vi "Datasheet Create Table Row.vi"(8 "error in (no error)":errorcluster, 9 "TDM Data":T2[](array[typedef]), 10 "Columns":T1[](array[typedef])) -> (0 "error out":errorcluster, 2 "Comma row":string, 3 "HTM Row":string)   [LabVIEW 2011]
uses:
  TDMS/TDMS File.ctl
  TDMS/TDMS Run.ctl
  TDMS/TDMS Channel (Sxx).ctl
  database/Fields/Field Record.ctl
  database/Fields/Field DataTypes.ctl
  database/Fields/Field NextItem.ctl
  Column Data.ctl
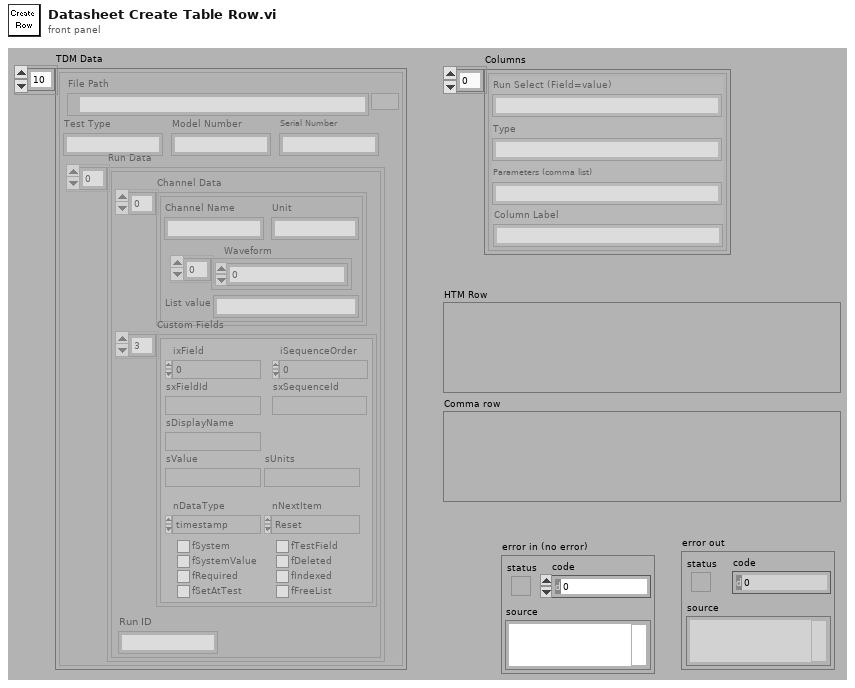
[diagram p1: front panel]
types:
  T1 = typedef "Column Data.ctl" = cluster{"Run Select (Field=value)":string, "Type":string, "Parameters (comma list)":string, "Column Label":string}
  T2 = typedef "TDMS File.ctl" = cluster{"File Path":path, "Run Data":T3[], "Serial Number":string, "Model Number":string, "Test Type":string}
  T3 = typedef "TDMS Run.ctl" = cluster{"Channel Data":T4[], "Custom Fields":T5[], "Run ID":string}
  T4 = typedef "TDMS Channel (Sxx).ctl" = cluster{"Channel Name":string, "Waveform":dbl[], "Unit":string, "List value":string}
  T5 = typedef "Field Record.ctl" = cluster{"ixField":i32, "iSequenceOrder":i32, "sxFieldId":string, "sxSequenceId":string, "sDisplayName":string, "sValue":string, "sUnits":string, "nDataType":T6, "nNextItem":T7, "fSystem":bool, "fSystemValue":bool, "fRequired":bool, "fSetAtTest":bool, "fTestField":bool, "fDeleted":bool, "fIndexed":bool, "fFreeList":bool}
  T6 = typedef "Field DataTypes.ctl" = enum32{"text", "numeric", "list", "timestamp", "boolean"}
  T7 = typedef "Field NextItem.ctl" = enum32{"Reset", "Retain", "Auto-Increment"}
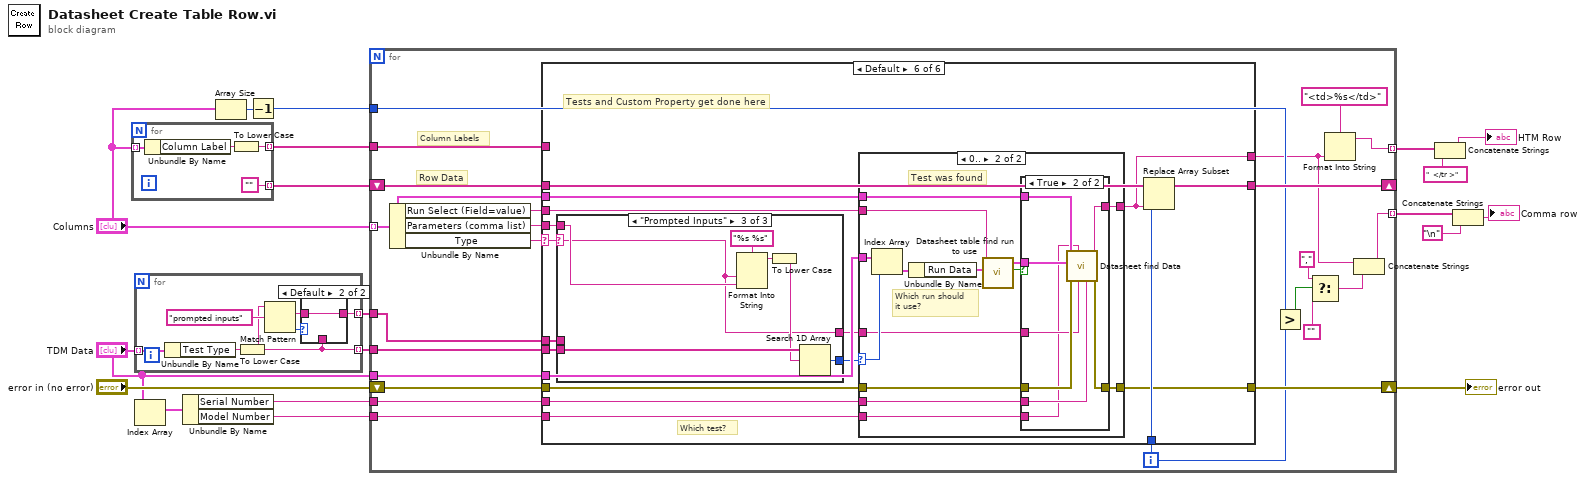
[diagram p0: block diagram]
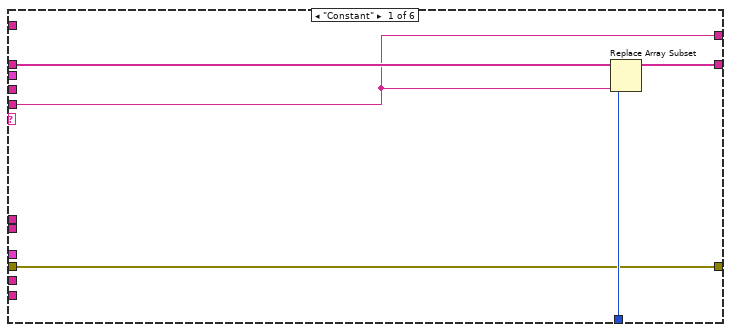
[diagram p3: hidden frame]
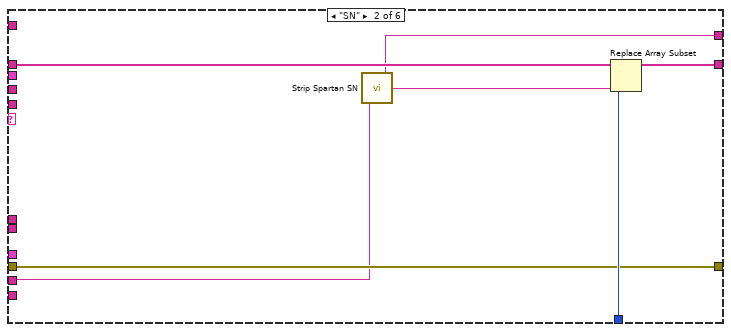
[diagram p4: hidden frame]
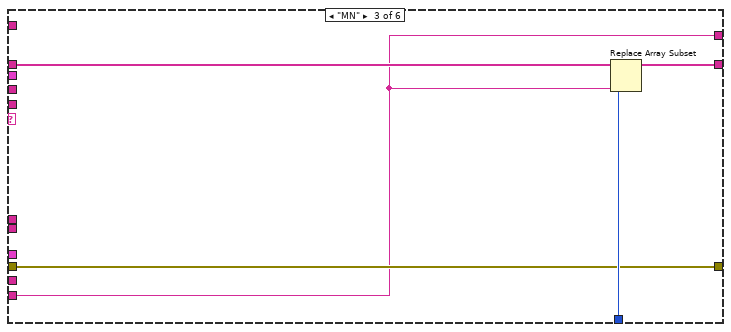
[diagram p5: hidden frame]
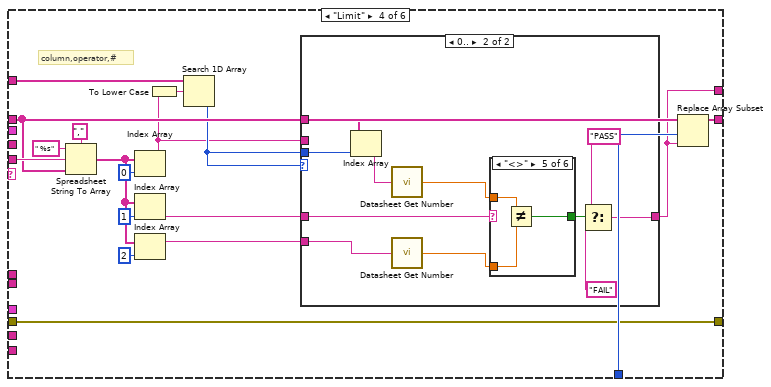
[diagram p6: hidden frame]
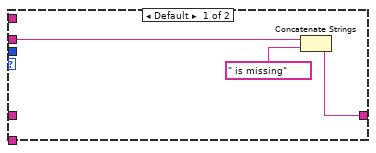
[diagram p7: hidden frame]
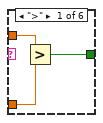
[diagram p8: hidden frame]
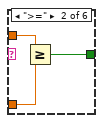
[diagram p9: hidden frame]
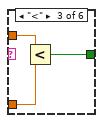
[diagram p10: hidden frame]
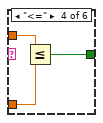
[diagram p11: hidden frame]
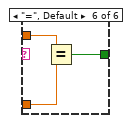
[diagram p12: hidden frame]
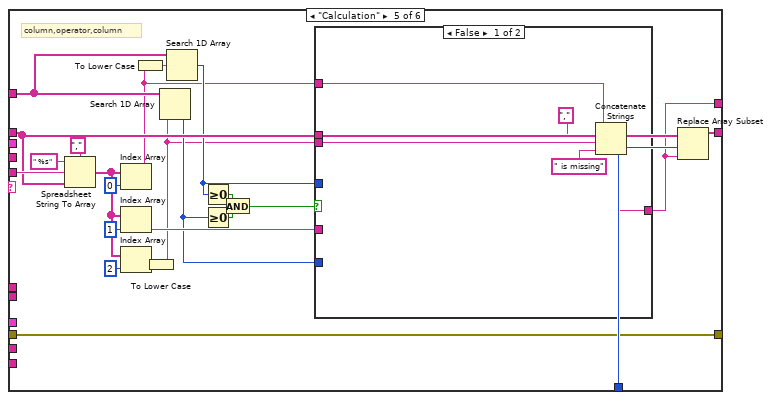
[diagram p13: hidden frame]
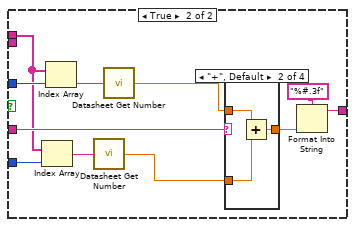
[diagram p14: hidden frame]
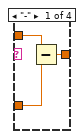
[diagram p15: hidden frame]
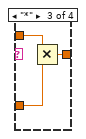
[diagram p16: hidden frame]
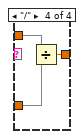
[diagram p17: hidden frame]
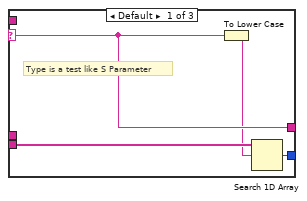
[diagram p18: hidden frame]
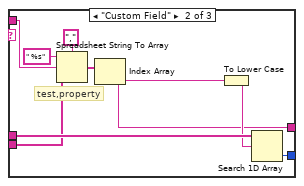
[diagram p19: hidden frame]
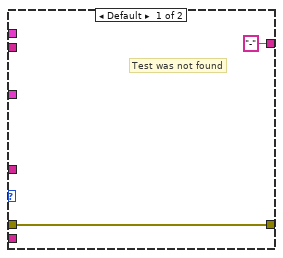
[diagram p20: hidden frame]
diagram:
  n1 = for {
    tunnel: "Columns" -> [w23] mode=indexing
    tunnel: [""] -> w16 mode=indexing
    tunnel: [w20] -> w3 mode=indexing
    n2 = Unbundle By Name(w23) -> ("Column Label"=w21:string)
    n3 = To Lower Case(string=w21) -> (all lower case string=w20:string)
  }
  n4 = for {
    tunnel: "TDM Data" -> [w30] mode=indexing
    tunnel: [w25] -> w17 mode=indexing
    tunnel: [w26] -> w1 mode=indexing
    n5 = Unbundle By Name(w30) -> ("Test Type"=w29:string)
    n6 = To Lower Case(string=w29) -> (all lower case string=w25:string)
    n7 = Match Pattern(string=w25, regular expression="prompted inputs") -> (match substring=w24:string, offset past match=w27:i32)  [unwired: 1 in, 2 out]
    n8 = case shown="Default" w27 {
      tunnel: [w31 w32] -> w26
      tunnel: w25 -> [w31 _]
      tunnel: w24 -> [_ w32]
      frame -1 {
      }
      frame Default {
      }
    }
  }
  n9 = Index Array(array="TDM Data") -> (element=w9:T2)  [unwired: 1 in]
  n10 = Unbundle By Name(w9) -> ("Serial Number"=w8:string, "Model Number"=w7:string)
  n11 = Array Size(array="Columns") -> (size(s)=w12:i32)
  n12 = Decrement(x=w12) -> (x-1=w5:i32)
  n13 = for {
    tunnel: "Columns" -> [w47] mode=indexing
    tunnel: "TDM Data" -> [w44]
    tunnel: w17 -> [w56]
    tunnel: w3 -> [w52]
    shift-right: [w48] -> _
    shift-left: w16 -> [w53]
    tunnel: [w51] -> w10 mode=indexing
    shift-right: [w45] -> w14
    shift-left: "error in (no error)" -> [w46]
    tunnel: w8 -> [w43]
    tunnel: w7 -> [w42]
    tunnel: w5 -> [w38]
    tunnel: [w36] -> w4 mode=indexing
    tunnel: w1 -> [w33]
    i -> [w34]
    # "Column Labels"
    # "Row Data"
    n14 = Unbundle By Name(w47) -> ("Run Select (Field=value)"=w55:string, "Parameters (comma list)"=w49:string, "Type"=w54:string)
    n15 = case shown="Default" w54 {
      selector: w54 -> [_ _ _ _ _ w183]
      tunnel: w56 -> [_ _ _ _ _ w174]
      tunnel: w44 -> [_ _ _ _ _ w190]
      tunnel: w55 -> [_ _ _ _ _ w189]
      tunnel: w53 -> [w61 w67 w72 w84 w134 w188]
      tunnel: w52 -> [_ _ _ w88 w136 _]
      tunnel: [w59 w62 w68 w78 w133 w185] -> w37
      tunnel: w49 -> [w59 _ _ w87 w143 w180]
      tunnel: w34 -> [w60 w66 w71 w90 w145 w186]
      tunnel: [w58 w65 w70 w89 w144 w187] -> w48
      tunnel: w47 -> [_ _ _ _ _ w184]
      tunnel: w46 -> [w57 w64 w69 w76 w131 w182]
      tunnel: [w57 w64 w69 w76 w131 w181] -> w45
      tunnel: w43 -> [_ w63 _ _ _ w178]
      tunnel: w42 -> [_ _ w68 _ _ w179]
      tunnel: w33 -> [_ _ _ _ _ w177]
      frame "Constant" {
        n16 = Replace Array Subset(array=w61, new element=w59, index=w60) -> (w58:string[])
      }
      frame "SN" {
        n17 = call "Strip Spartan SN.vi"("SN 2"=w63) -> ("SN"=w62:string)
        n18 = Replace Array Subset(array=w67, new element=w62, index=w66) -> (w65:string[])
      }
      frame "MN" {
        n19 = Replace Array Subset(array=w72, new element=w68, index=w71) -> (w70:string[])
      }
      frame "Limit" {
        # "column,operator,#"
        n20 = Spreadsheet String To Array(delimiter (Tab)=",", format string=" %s" ("delimiter (Tab)"), spreadsheet string=w87, array type (2D Dbl)=w84) -> (array=w83:string[])
        n21 = Index Array(array=w83, index=0) -> (element=w73:string)
        n22 = Index Array(array=w83, index=1) -> (element=w80:string)
        n23 = Index Array(array=w83, index=2) -> (element=w79:string)
        n24 = To Lower Case(string=w73) -> (all lower case string=w75:string)
        n25 = Search 1D Array(1D array=w88, element=w75) -> (index of element=w74:i32)  [unwired: 1 out]
        n26 = case shown="0.." w74 {
          tunnel: w84 -> [_ w104]
          tunnel: w74 -> [_ w103]
          tunnel: w80 -> [_ w102]
          tunnel: w79 -> [_ w100]
          tunnel: [w92 w95] -> w78
          tunnel: w73 -> [w93 _]
          frame Default {
            n27 = Concatenate Strings(w93, " is missing" ("format string")) -> (w92:string)
          }
          frame 0.. {
            n28 = Index Array(array=w104, index=w103) -> (element=w101:string)
            n29 = call "Datasheet Get Number.vi"("String"=w101) -> ("Numeric"=w99:dbl)
            n30 = call "Datasheet Get Number.vi"("String"=w100) -> ("Numeric"=w98:dbl)
            n31 = case shown="\"<>\"" w102 {
              tunnel: w99 -> [w107 w110 w113 w116 w119 w122]
              tunnel: w98 -> [w106 w109 w112 w115 w118 w121]
              tunnel: [w105 w108 w111 w114 w117 w120] -> w97
              frame ">" {
                n32 = Greater?(x=w107, y=w106) -> (0:w105:bool)
              }
              frame ">=" {
                n33 = Greater Or Equal?(x=w110, y=w109) -> (x >= y?=w108:bool)
              }
              frame "<" {
                n34 = Less?(x=w113, y=w112) -> (x < y?=w111:bool)
              }
              frame "<=" {
                n35 = Less Or Equal?(x=w116, y=w115) -> (x <= y?=w114:bool)
              }
              frame "<>" {
                n36 = Not Equal?(x=w119, y=w118) -> (x != y?=w117:bool)
              }
              frame "=", Default {
                n37 = Equal?(x=w122, y=w121) -> (x = y?=w120:bool)
              }
            }
            n38 = Select(t="PASS" ("format string"), s=w97, f="FAIL" ("format string")) -> (s? t:f=w95:string)
          }
        }
        n39 = Replace Array Subset(array=w84, new element=w78, index=w90) -> (w89:string[])
      }
      frame "Calculation" {
        # "column,operator,column"
        n40 = Spreadsheet String To Array(delimiter (Tab)=",", format string=" %s" ("delimiter (Tab)"), spreadsheet string=w143, array type (2D Dbl)=w134) -> (array=w140:string[])
        n41 = Index Array(array=w140, index=0) -> (element=w124:string)
        n42 = Index Array(array=w140, index=1) -> (element=w137:string)
        n43 = Index Array(array=w140, index=2) -> (element=w135:string)
        n44 = To Lower Case(string=w124) -> (all lower case string=w130:string)
        n45 = To Lower Case(string=w135) -> (all lower case string=w123:string)
        n46 = Search 1D Array(1D array=w136, element=w123) -> (index of element=w126:i32)  [unwired: 1 out]
        n47 = Search 1D Array(1D array=w136, element=w130) -> (index of element=w127:i32)  [unwired: 1 out]
        n48 = Greater Or Equal To 0?(x=w127) -> (x >= 0?=w129:bool)
        n49 = Greater Or Equal To 0?(x=w126) -> (x >= 0?=w128:bool)
        n50 = And(x=w129, y=w128) -> (x .and. y?=w125:bool)
        n51 = case shown="False" w125 {
          tunnel: w137 -> [_ w161]
          tunnel: w127 -> [_ w160]
          tunnel: w134 -> [_ w159]
          tunnel: w126 -> [_ w158]
          tunnel: [w149 w156] -> w133
          tunnel: w124 -> [w148 _]
          tunnel: w123 -> [w147 _]
          frame False {
            n52 = Concatenate Strings(w148, "," ("format string"), w147, " is missing" ("format string")) -> (w149:string)
          }
          frame True {
            n53 = Index Array(array=w159, index=w158) -> (element=w152:string)
            n54 = Index Array(array=w159, index=w160) -> (element=w154:string)
            n55 = call "Datasheet Get Number.vi"("String"=w152) -> ("Numeric"=w151:dbl)
            n56 = call "Datasheet Get Number.vi"("String"=w154) -> ("Numeric"=w153:dbl)
            n57 = case shown="\"+\", Default" w161 {
              tunnel: w153 -> [w164 w167 w170 w173]
              tunnel: w151 -> [w163 w166 w169 w172]
              tunnel: [w162 w165 w168 w171] -> w157
              frame "-" {
                n58 = Subtract(x=w164, y=w163) -> (x-y=w162:dbl)
              }
              frame "+", Default {
                n59 = Add(x=w167, y=w166) -> (x+y=w165:dbl)
              }
              frame "*" {
                n60 = Multiply(x=w170, y=w169) -> (x*y=w168:dbl)
              }
              frame "/" {
                n61 = Divide(x=w173, y=w172) -> (x/y=w171:dbl)
              }
            }
            n62 = Format Into String(format string="%#.3f", w157) -> (resulting string=w156:string)  [unwired: 2 in, 1 out]
          }
        }
        n63 = Replace Array Subset(array=w134, new element=w133, index=w145) -> (w144:string[])
      }
      frame Default {
        # "Which test?"
        # "Tests and Custom Property get done here"
        n64 = case shown="\"Prompted Inputs\"" w183 {
          selector: w183 -> [w194 _ w204]
          tunnel: w180 -> [_ w201 w205]
          tunnel: w177 -> [_ w199 _]
          tunnel: [w193 w198 w208] -> w176
          tunnel: [w194 w196 w204] -> w175
          tunnel: w174 -> [w192 w195 w207]
          frame Default {
            # "Type is a test like S Parameter"
            n65 = To Lower Case(string=w194) -> (all lower case string=w191:string)
            n66 = Search 1D Array(1D array=w192, element=w191) -> (index of element=w193:i32)  [unwired: 1 out]
          }
          frame "Custom Field" {
            # "test,property"
            n67 = Spreadsheet String To Array(delimiter (Tab)=",", format string=" %s" ("delimiter (Tab)"), spreadsheet string=w201, array type (2D Dbl)=w195) -> (array=w200:string[])
            n68 = Index Array(array=w200) -> (element=w196:string)  [unwired: 1 in]
            n69 = To Lower Case(string=w196) -> (all lower case string=w197:string)
            n70 = Search 1D Array(1D array=w199, element=w197) -> (index of element=w198:i32)  [unwired: 1 out]
          }
          frame "Prompted Inputs" {
            n71 = Format Into String(format string="%s %s", w204, w205) -> (resulting string=w209:string)  [unwired: 2 in, 1 out]
            n72 = To Lower Case(string=w209) -> (all lower case string=w206:string)
            n73 = Search 1D Array(1D array=w207, element=w206) -> (index of element=w208:i32)  [unwired: 1 out]
          }
        }
        n74 = case shown="0.." w176 {
          selector: w176 -> [_ w225]
          tunnel: w190 -> [_ w226]
          tunnel: w189 -> [_ w223]
          tunnel: ["-" ("format string") w219] -> w185
          tunnel: w184 -> [_ w221]
          tunnel: w182 -> [w211 w217]
          tunnel: [w211 w216] -> w181
          tunnel: w179 -> [_ w213]
          tunnel: w178 -> [_ w215]
          tunnel: w175 -> [_ w214]
          frame Default {
            # "Test was not found"
          }
          frame 0.. {
            # "Which run should\nit use?"
            # "Test was found"
            n75 = Index Array(array=w226, index=w225) -> (element=w224:T2)
            n76 = Unbundle By Name(w224) -> ("Run Data"=w222:T3[])
            n77 = call "Datasheet table find run to use.vi"("Run Data"=w222, "Run Select (Field=value)"=w223) -> ("Found Run?"=w218:bool, "Run Information"=w220:T3)  [unwired: 8 out]
            n78 = case shown="True" w218 {
              tunnel: w221 -> [_ w236]
              tunnel: w220 -> [_ w235]
              tunnel: ["Missing Run" ("format string") w234] -> w219
              tunnel: w217 -> [w227 w233]
              tunnel: [w227 w232] -> w216
              tunnel: w215 -> [_ w231]
              tunnel: w214 -> [_ w230]
              tunnel: w213 -> [_ w229]
              frame False {
              }
              frame True {
                n79 = call "Datasheet find Data.vi"("SN"=w231, "Test Type"=w230, "MN"=w229, "error in (no error)"=w233, "Run Information"=w235, "Column Data"=w236) -> ("error out"=w232:errorcluster, "Column Item"=w234:string)  [unwired: 4 out]
              }
            }
          }
        }
        n80 = Replace Array Subset(array=w188, new element=w185, index=w186) -> (w187:string[])
      }
    }
    n81 = Greater?(x=w38, y=w34) -> (0:w41:bool)
    n82 = Select(t="," ("format string"), s=w41, f="") -> (s? t:f=w39:string)
    n83 = Format Into String(format string="<td>%s</td>", w37) -> (resulting string=w51:string)  [unwired: 2 in, 1 out]
    n84 = Concatenate Strings(w37, w39) -> (w36:string)
  }
  "error out" <- w14
  n85 = Concatenate Strings(w10, "  </tr >" ("format string")) -> (→"HTM Row":string)
  n86 = Concatenate Strings(w4, "\n") -> (→"Comma row":string)
